vi "Activate Reservoir.vi"(8 "error in (no error)":errorcluster, 10 "SignalCluster in":T1, 11 "Queue in":refnum<queue>) -> (0 "error out":errorcluster, 3 "SignalCluster out":T1)   [LabVIEW 2013, in "main.lvlib"]
uses:
  main.lvlib
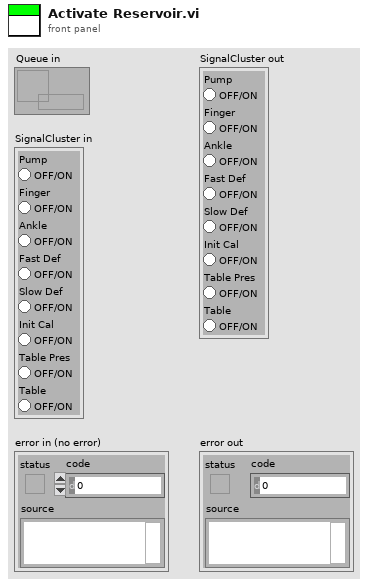
[diagram p1: front panel]
types:
  T1 = cluster{"Pump":bool, "Finger":bool, "Ankle":bool, "Fast Def":bool, "Slow Def":bool, "Init Cal":bool, "Table Pres":bool, "Table":bool}
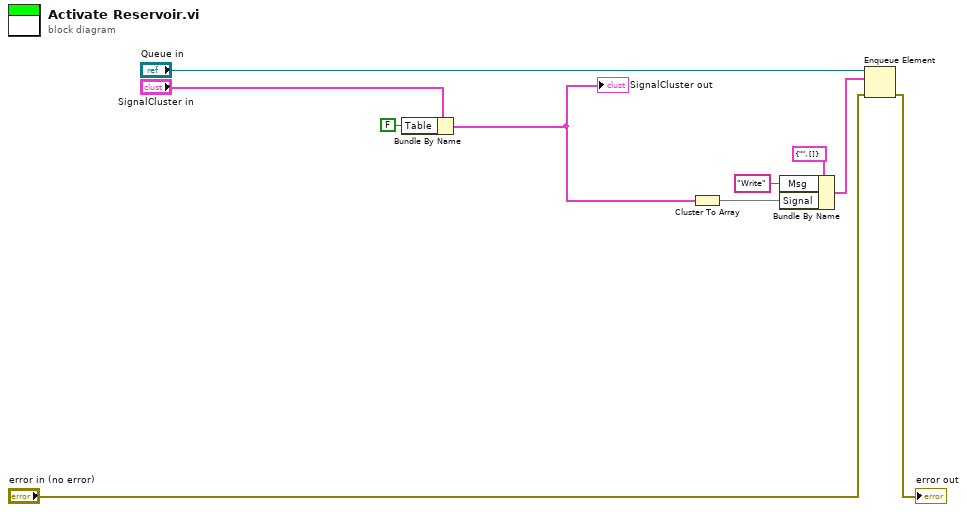
[diagram p0: block diagram]
diagram:
  n1 = Bundle By Name(cluster="SignalCluster in", "Table"=FALSE ("Fast Def")) -> (w7:T1)
  "SignalCluster out" <- w7
  n2 = Cluster To Array(cluster=w7) -> (array=w3:bool[])
  n3 = Bundle By Name(cluster=cluster{"Msg":string, "Signal":bool[]} {"Msg"="", "Signal"=[]} ("element"), "Msg"="Write", "Signal"=w3) -> (w5:cluster{"Msg":string, "Signal":bool[]})
  n4 = Enqueue Element(queue="Queue in", element=w5, error in (no error)="error in (no error)") -> (error out=→"error out":errorcluster)  [unwired: 1 in, 2 out]
